vi "Handle Value Change.vi"(5 "VolatusAPI":refnum<class "VolatusAPI.lvclass">, 7 "CtlRef":refnum<vi>, 8 "error in (no error)":errorcluster, 9 "NewVal":variant, 10 "OldVal":variant, 11 "GuiLinkButton in":refnum<class "GuiLinkButton.lvclass">) -> (0 "error out":errorcluster, 3 "GuiLinkButton out":refnum<class "GuiLinkButton.lvclass">)   [LabVIEW 2020, in "VolatusGUIElements.lvlib" / "GuiLinkButton.lvclass"]
uses:
  GuiLinkButton.lvclass
  Volatus/VolatusAPI/VolatusAPI.lvclass
  GuiLinkButton.lvclass/GuiLinkButton.ctl
  Volatus/GUI Manager Identity/GUI Manager Identity.lvclass
  C:/dev/lv20CE/relink/lv-volatus/Volatus/GUI Manager Identity/GUI Manager Identity.lvclass
  C:/dev/lv20CE/relink/lv-volatus/Volatus/Identity/Identity.lvclass
  Volatus/MessageQ/MessageQ.lvclass
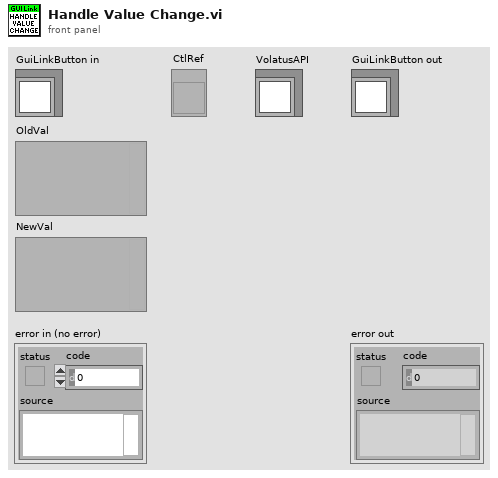
[diagram p1: front panel]
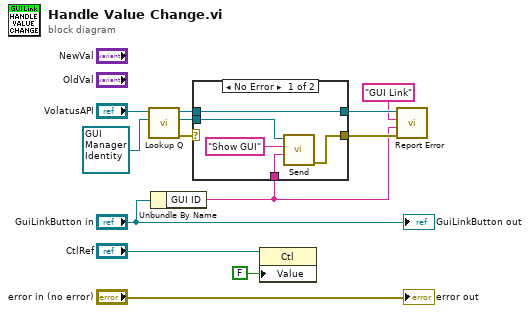
[diagram p0: block diagram]
diagram:
  n1 = call "Lookup Q.vi"("Identity"=refnum<class "GUI Manager Identity.lvclass"> refnum ("VolatusGUI:GUI Manager Identity.lvclass"), "VolatusAPI in"="VolatusAPI") -> ("error out"=w8:errorcluster, "MessageQ"=w6:refnum<class "MessageQ.lvclass">, "VolatusAPI out"=w7:refnum<class "VolatusAPI.lvclass">)  [unwired: 7 in]
  n2 = Unbundle By Name("GuiLinkButton in") -> ("GUI ID"=w1:string)
  n3 = case shown="No Error" w8 {
    selector: w8 -> [_ w20]
    tunnel: w7 -> [w14 w19]
    tunnel: w6 -> [w18 _]
    tunnel: [w15 w20] -> w4
    tunnel: [w14 w19] -> w5
    tunnel: w1 -> [w16 _]
    frame No Error {
      n4 = call "Send.vi"("Data"=w16, "ID"="Show GUI", "MessageQ in"=w18) -> ("error out"=w15:errorcluster)  [unwired: 7 in, 1 out]
    }
    frame Error {
    }
  }
  n5 = property class="Ctl"(reference="CtlRef", "Value"=FALSE) -> ()  [unwired: 1 in, 2 out]
  n6 = call "Report Error.vi"("error in (no error)"=w4, "Message"=w1, "Context"="GUI Link", "VolatusAPI in"=w5) -> ()  [unwired: 6 in, 2 out]
  "error out" <- "error in (no error)"
  "GuiLinkButton out" <- "GuiLinkButton in"
